vi "onExecuteJob.vi"(8 "error in (no error)":errorcluster, 10 "stdin":string, 11 "Job.SingleFileCopy in":refnum<class "Job.BuildSpec.lvclass">) -> (0 "error out":errorcluster, 1 "exception":i32, 2 "stdout":string, 3 "Job.SingleFileCopy":refnum<class "Job.BuildSpec.lvclass">)   [LabVIEW 2013, in "Job.BuildSpec.lvclass"]
uses:
  Job.BuildSpec.lvclass
  BuildSpec Job Configuration -- cluster.ctl
  Job.BuildSpec.lvclass/Job.BuildSpec.ctl
  <vilib>/LabVIEW Open Source Project/Cron Scheduler/Job/Job.lvclass
  <vilib>/addons/_JKI.lib/Serialization/JSON/JKI JSON Serialization.lvlib
panel:
  # "RUNNING A JOB"
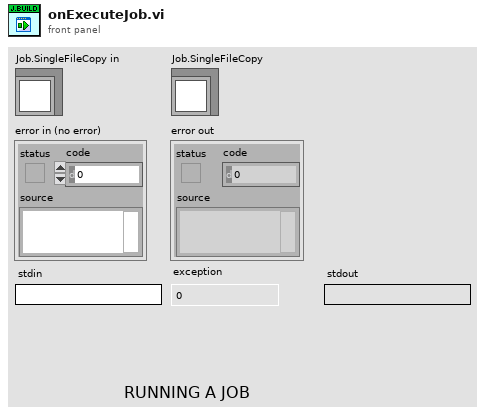
[diagram p1: front panel]
types:
  T1 = typedef "Job.BuildSpec.lvclass/BuildSpec Job Configuration -- cluster.ctl" = cluster{"Project Path":path, "Build Name":string, "Target":string, "Clean":bool, "Deploy":bool}
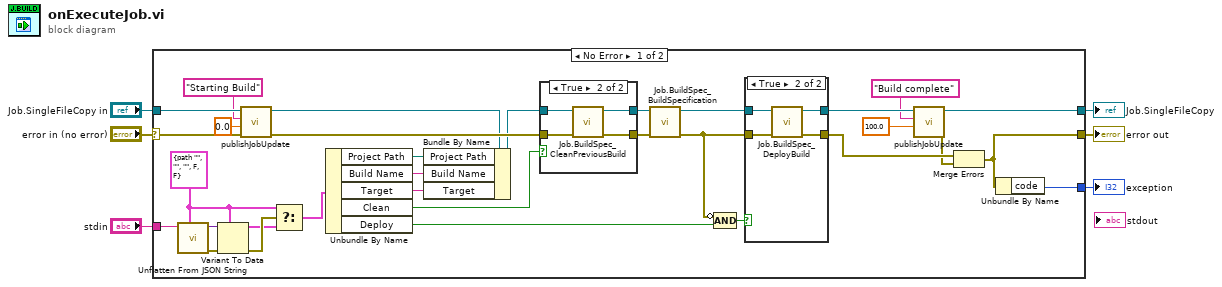
[diagram p0: block diagram]
diagram:
  n1 = case shown="No Error" "error in (no error)" {
    selector: "error in (no error)" -> [w35 w52]
    tunnel: "stdin" -> [w33 _]
    tunnel: "Job.SingleFileCopy in" -> [w38 w51]
    tunnel: [w12 w52] -> w4
    tunnel: [w18 w51] -> w2
    tunnel: [w34 _] -> w1
    frame No Error {
      w28 = T1 {"Project Path"=path "", "Build Name"="", "Target"="", "Clean"=FALSE, "Deploy"=FALSE} ("FileCopy Job Config")
      n2 = call <vilib>:"Unflatten From JSON String.vi"("Type and Defaults"=w28, "JSON String"=w33) -> ("error out"=w32:errorcluster, "Variant"=w31:variant)  [unwired: 8 in]
      n3 = Variant To Data(error in=w32, type=w28, Variant=w31) -> (data=w29:T1, error out=w30:errorcluster)
      n4 = call <vilib>:"publishJobUpdate.vi"("error in (no error)"=w35, "% Complete (NaN if unknown)"=0.0, "Status Message"="Starting Build", "Job in"=w38) -> ("error out"=w24:errorcluster, "Job out"=w11:refnum<class "Job.BuildSpec.lvclass">)  [unwired: 6 in]
      n5 = Select(t=w28, s=w30, f=w29) -> (s? t:f=w27:T1)
      n6 = Unbundle By Name(w27) -> ("Project Path"=w9:path, "Build Name"=w8:string, "Target"=w7:string, "Clean"=w23:bool, "Deploy"=w26:bool)
      n7 = Bundle By Name(cluster=w11, "Project Path"=w9, "Build Name"=w8, "Target"=w7) -> (w10:refnum<class "Job.BuildSpec.lvclass">)
      n8 = case shown="True" w23 {
        tunnel: w24 -> [w39 w44]
        tunnel: w10 -> [w40 w43]
        tunnel: [w40 w42] -> w22
        tunnel: [w39 w41] -> w21
        frame False {
        }
        frame True {
          n9 = call "Job.BuildSpec_CleanPreviousBuild.vi"("error in (no error)"=w44, "Job.BuildSpec in"=w43) -> ("error out"=w41:errorcluster, "Job.BuildSpec out"=w42:refnum<class "Job.BuildSpec.lvclass">)  [unwired: 8 in]
        }
      }
      n10 = call "Job.BuildSpec_BuildSpecification.vi"("error in (no error)"=w21, "Job.BuildSpec in"=w22) -> ("error out"=w15:errorcluster, "Job.BuildSpec out"=w20:refnum<class "Job.BuildSpec.lvclass">)  [unwired: 8 in]
      n11 = Compound Arithmetic op=AND(invert w15, w26) -> (w25:bool)
      n12 = case shown="True" w25 {
        tunnel: [w45 w47] -> w14
        tunnel: w20 -> [w46 w50]
        tunnel: [w46 w49] -> w17
        tunnel: w15 -> [w45 w48]
        frame False {
        }
        frame True {
          n13 = call "Job.BuildSpec_DeployBuild.vi"("error in (no error)"=w48, "Job.BuildSpec in"=w50) -> ("error out"=w47:errorcluster, "Job.BuildSpec out"=w49:refnum<class "Job.BuildSpec.lvclass">)  [unwired: 8 in]
        }
      }
      n14 = call <vilib>:"publishJobUpdate.vi"("% Complete (NaN if unknown)"=100.0, "Status Message"="Build complete", "Job in"=w17) -> ("error out"=w13:errorcluster, "Job out"=w18:refnum<class "Job.BuildSpec.lvclass">)  [unwired: 7 in]
      n15 = Merge Errors(w14, w13) -> (w12:errorcluster)
      n16 = Unbundle By Name(w12) -> ("code"=w34:i32)
    }
    frame Error {
    }
  }
  "error out" <- w4
  "Job.SingleFileCopy" <- w2
  "exception" <- w1
